vi "Runner.vi"(8 "error in (no error)":errorcluster, 10 "Runnable":refnum<class "Runnable.lvclass">, 11 "Parallell Test Runner In":refnum<class "Parallell Test Runner.lvclass">) -> (0 "error out":errorcluster)   [LabVIEW 2020, in "Parallell Test Runner.lvclass"]
uses:
  Parallell Test Runner.lvclass
  Runnable.lvclass
  Core/Result/Result.ctl
  Core/Result/Status.ctl
  Core/Result/Type.ctl
  Parallell Test Runner.lvclass/Parallell Test Runner.ctl
  <vilib>/AdvancedString/Delimited String to 1D String Array.vi
  <vilib>/AdvancedString/1D String Array to Delimited String.vi
  Result Observer/Result Observer.lvclass
  Execute Suite.vi
  LUnit Test Suite.lvclass
  Core/Result/Result.lvlib
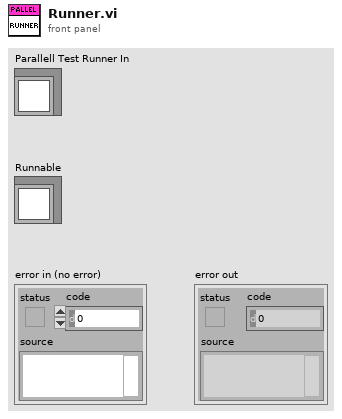
[diagram p1: front panel]
types:
  T1 = typedef "Result.lvlib/Result.ctl" = cluster{"Name":string, "Description":string, "Status":T2, "Result Type":T3, "Execution Time":dbl, "Data":cluster{"Expected":variant, "Actual":variant, "Delta":variant}}
  T2 = typedef "Result.lvlib/Status.ctl" = enum16{"", "Passed", "Failed", "Error", "Skipped", "Setup Error", "Broken", "Teardown Error"}
  T3 = typedef "Result.lvlib/Type.ctl" = enum16{"Test Case", "Test Suite", "Test Run", "Pass", "Fail", "Skip", "Pass if", "Fail if", "Pass if Error", "Fail if Error", "Pass if Equal", "Fail if Equal"}
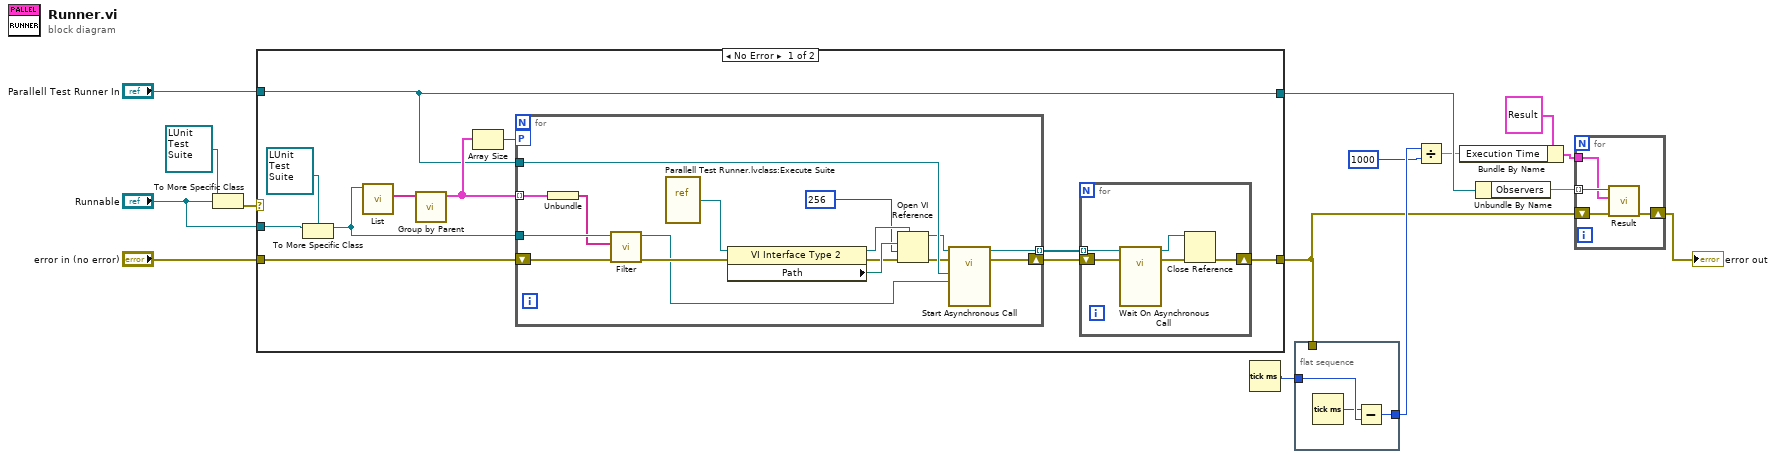
[diagram p0: block diagram]
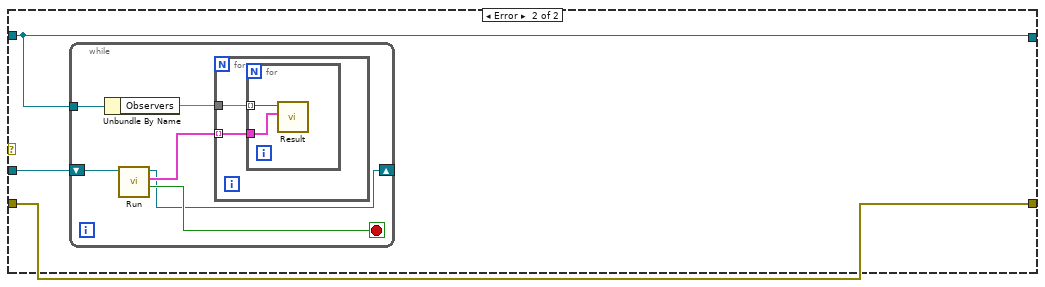
[diagram p2: hidden frame]
diagram:
  n1 = To More Specific Class(target class="Runnable", reference=refnum<class "LUnit Test Suite.lvclass"> refnum ("target class")) -> (error out=w9:errorcluster)  [unwired: 1 in, 1 out]
  n2 = case shown="No Error" w9 {
    tunnel: "Parallell Test Runner In" -> [w19 w50]
    tunnel: "error in (no error)" -> [w23 w48]
    tunnel: [w22 w48] -> w6
    tunnel: [w19 w50] -> w8
    tunnel: "Runnable" -> [w18 w49]
    frame No Error {
      n3 = To More Specific Class(target class=refnum<class "LUnit Test Suite.lvclass"> refnum, reference=w18) -> (specific class reference=w16:refnum<class "LUnit Test Suite.lvclass">)  [unwired: 1 in, 1 out]
      n4 = call "List.vi"("LUnit Test Suite In"=w16) -> ("List of Runnables"=w26:string[])  [unwired: 9 in, 1 out]
      n5 = call "Group by Parent.vi"("List of Runnables"=w26) -> ("Methods"=w21:cluster{"Methods":string[]}[])  [unwired: 10 in]
      n6 = Array Size(array=w21) -> (size(s)=w20:i32)
      n7 = for {
        tunnel: w16 -> [w42]
        shift-right: [w41] -> w25
        shift-left: w23 -> [w40]
        tunnel: w21 -> [w35] mode=indexing
        tunnel: [w37] -> w24 mode=indexing
        workers-P: w20 -> [_]
        tunnel: w19 -> [w36]
        n8 = Unbundle(w35) -> ("Methods"=w34:string[])
        n9 = call "Filter.vi"("error in (no error)"=w40, "Selected Runnables"=w34, "LUnit Test Suite In"=w42) -> ("error out"=w39:errorcluster, "LUnit Test Suite Out"=w38:refnum<class "LUnit Test Suite.lvclass">)  [unwired: 7 in]
        n10 = vi-ref "Parallell Test Runner.lvclass:Execute Suite.vi"() -> (w33:refnum<vi>)
        n11 = property class="VI Interface Type 2"(reference=w33, error in=w39) -> (reference out=w31:refnum<vi>, error out=w30:errorcluster, "Path"=w32:path)
        n12 = Open VI Reference(type specifier VI Refnum (for type only)=w31, vi path=w32, options=256, error in (no error)=w30) -> (vi reference=w29:refnum<vi>, error out=w28:errorcluster)  [unwired: 2 in]
        n13 = call-by-ref "Start Asynchronous Call"(reference=w29, error in=w28, "Runnable"=w38, "Parallell Test Runner In"=w36) -> (reference out=w37:refnum<vi>, error out=w41:errorcluster)  [unwired: 10 in]
      }
      n14 = for {
        shift-right: [w46] -> w22
        shift-left: w25 -> [w47]
        tunnel: w24 -> [w45] mode=indexing
        n15 = call-by-ref "Wait On Asynchronous Call"(reference=w45, error in=w47) -> (reference out=w44:refnum<vi>, error out=w43:errorcluster)  [unwired: 12 in]
        n16 = Close Reference(reference=w44, error in (no error)=w43) -> (error out=w46:errorcluster)
      }
    }
    frame Error {
      n17 = while {
        shift-right: [w54] -> _
        shift-left: w49 -> [w53]
        tunnel: w50 -> [w52]
        stop <- w55 stop-if-true
        n18 = Unbundle By Name(w52) -> ("Observers"=w51:set{refnum<class "Result Observer.lvclass">})
        n19 = call-dynamic "Run.vi"("Runnable In"=w53) -> ("Done?"=w55:bool, "Results"=w56:T1[], "Runnable Out"=w54:refnum<class "Runnable.lvclass">)  [unwired: 7 in, 1 out]
        n20 = for {
          tunnel: w56 -> [w57] mode=indexing
          tunnel: w51 -> [w58]
          n21 = for {
            tunnel: w58 -> [w60] mode=indexing
            tunnel: w57 -> [w59]
            n22 = call-dynamic "Result.vi"("Result"=w59, "Result Observer In"=w60) -> ()  [unwired: 9 in, 1 out]
          }
        }
      }
    }
  }
  n23 = Tick Count (ms)() -> (millisecond timer value=w12:u32)
  n24 = flat-sequence {
    tunnel: w12 -> [w63]
    tunnel: [w62] -> w11
    tunnel: w6 -> [_]
    frame #0 {
      n25 = Tick Count (ms)() -> (millisecond timer value=w61:u32)
      n26 = Subtract(x=w61, y=w63) -> (x-y=w62:u32)
    }
  }
  n27 = Divide(x=w11, y=u32 1000) -> (x/y=w5:dbl)
  n28 = Bundle By Name(cluster=T1 {"Name"="", "Description"="", "Status"=enum."Passed", "Result Type"=enum."Test Run", "Execution Time"=0.0, "Data"={"Expected"=variant, "Actual"=variant, "Delta"=variant}} ("Result"), "Execution Time"=w5) -> (w2:T1)
  n29 = Unbundle By Name(w8) -> ("Observers"=w4:set{refnum<class "Result Observer.lvclass">})
  n30 = for {
    tunnel: w4 -> [w67] mode=indexing
    tunnel: w2 -> [w66]
    shift-right: [w64] -> w13
    shift-left: w6 -> [w65]
    n31 = call-dynamic "Result.vi"("error in (no error)"=w65, "Result"=w66, "Result Observer In"=w67) -> ("error out"=w64:errorcluster)  [unwired: 8 in]
  }
  "error out" <- w13
